vi "新FPGA ENC.vi"() -> ()   [LabVIEW 2017]
panel:
  in  "Reset ENC":bool
  out "ENC":i32
  in  "停止":bool
  in  "B":bool
  in  "A":bool
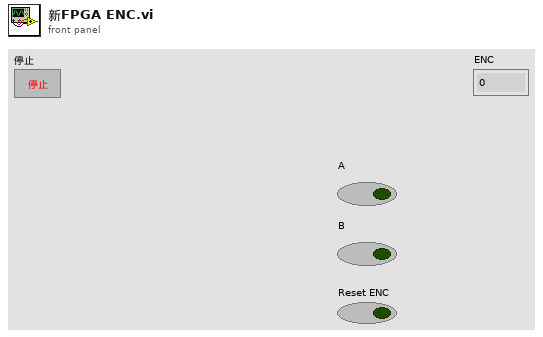
[diagram p1: front panel]
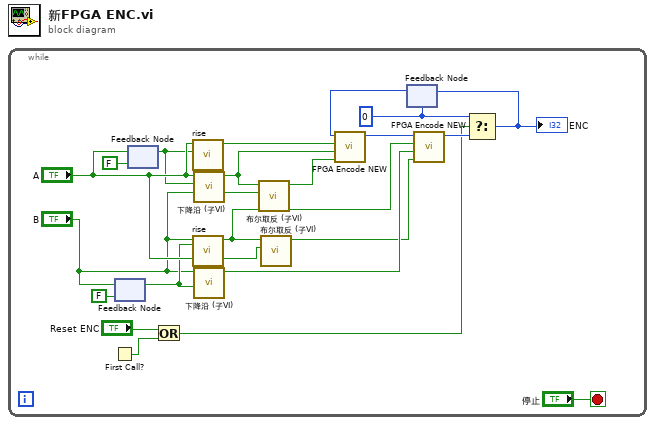
[diagram p0: block diagram]
diagram:
  n1 = while {
    stop <- "停止" stop-if-true
    w5 = 0
    n2 = First Call?() -> (First Call?: T/F=w2:bool)
    n3 = feedback #1(FALSE ("B")) -> (w10:bool)
    n4 = feedback-in #1("B") -> ()
    n5 = feedback-in #2("A") -> ()
    n6 = feedback #2(FALSE ("A")) -> (w11:bool)
    n7 = Or(x="Reset ENC", y=w2) -> (x .or. y?=w1:bool)
    n8 = call "rise.vi"("Last Signal"=w11, "Signal"="A") -> ("Count?"=w20:bool)  [unwired: 9 in]
    n9 = call "rise.vi"("Last Signal"=w10, "Signal"="B") -> ("Count?"=w15:bool)  [unwired: 9 in]
    n10 = call "下降沿 (子VI).vi"("Last Signal"=w11, "Signal"="A") -> ("Down?"=w19:bool)  [unwired: 9 in]
    n11 = call "下降沿 (子VI).vi"("Last Signal"=w10, "Signal"="B") -> ("Down?"=w14:bool)  [unwired: 9 in]
    n12 = call "布尔取反 (子VI).vi"("Signal"="B", "Enable¿"=w19) -> ("Output"=w18:bool)  [unwired: 9 in]
    n13 = call "布尔取反 (子VI).vi"("Signal"="A", "Enable¿"=w15) -> ("Output"=w13:bool)  [unwired: 9 in]
    n14 = feedback #3(w5) -> (w17:i32)
    n15 = call "FPGA Encode NEW .vi"("Direction"=w18, "Down"=w19, "Rise"=w20, "ENC"=w17) -> ("ENC+"=w16:i32)  [unwired: 7 in]
    n16 = call "FPGA Encode NEW .vi"("Direction"=w13, "Down"=w14, "Rise"=w15, "ENC"=w16) -> ("ENC+"=w7:i32)  [unwired: 7 in]
    n17 = Select(t=w5, s=w1, f=w7) -> (s? t:f=w6:i32)
    "ENC" <- w6
    n18 = feedback-in #3(w6) -> ()
  }
